vi "unmarshalling.vi"(7 "Type":variant, 8 "error in (no error)":errorcluster, 10 "JSON String":string, 11 "Serializer":refnum<class "Serializer.JDP-JSON.lvclass">) -> (0 "error out":errorcluster, 2 "Variant":variant, 3 "Serializer out":refnum<class "Serializer.JDP-JSON.lvclass">)   [LabVIEW 2019, in "OpenSerializer.JDP-JSON.lvlib" / "Serializer.JDP-JSON.lvclass"]
uses:
  Serializer.JDP-JSON.lvclass
  <vilib>/JDP Science/JSONtext/JSONtext.lvlib
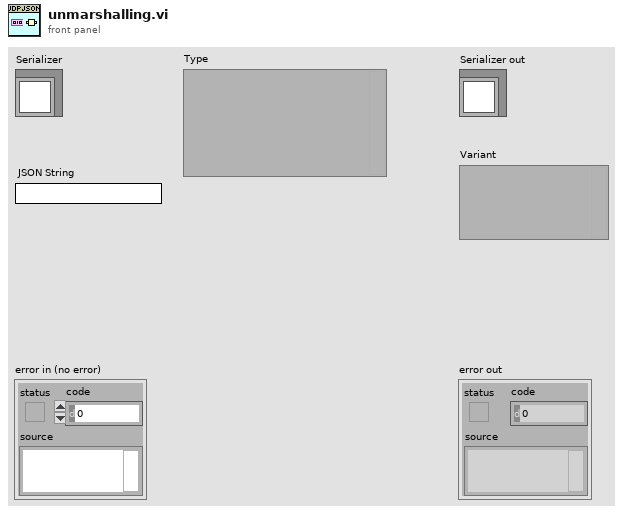
[diagram p1: front panel]
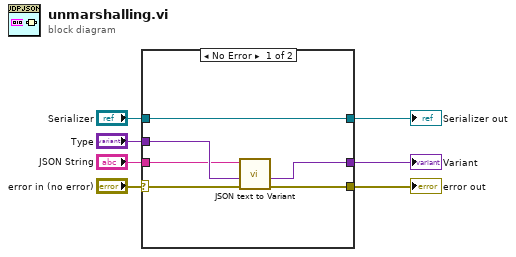
[diagram p0: block diagram]
diagram:
  n1 = case shown="No Error" "error in (no error)" {
    selector: "error in (no error)" -> [w10 w15]
    tunnel: "Serializer" -> [w13 w16]
    tunnel: "JSON String" -> [w11 _]
    tunnel: [w13 w16] -> w5
    tunnel: [w9 w15] -> w4
    tunnel: [w8 w14] -> w3
    tunnel: "Type" -> [w12 w14]
    frame No Error {
      n2 = call <vilib>:"JSON text to Variant.vi"("error in (no error)"=w10, "Data Type"=w12, "JSON"=w11) -> ("error out"=w9:errorcluster, "Variant out"=w8:variant)  [unwired: 7 in]
    }
    frame Error {
    }
  }
  "error out" <- w4
  "Serializer out" <- w5
  "Variant" <- w3
